vi "shoot boiler.vi"(7 "go":bool, 8 "error out":errorcluster, 11 "RobotDriveDevRef":T1={"DevStatus"={"status"=FALSE, "code"=0, "source"=""}, "Motors[]"=[], "Square Inputs"=FALSE, "Max Output"=1.0}) -> (0 "error out 2":errorcluster, 3 "RobotDriveDevRef 2":T1={"DevStatus"={"status"=FALSE, "code"=0, "source"=""}, "Motors[]"=[], "Square Inputs"=FALSE, "Max Output"=1.0})   [LabVIEW 2016]
uses:
  <vilib>/Rock Robotics/WPI/RobotDrive/WPI_RobotDriveDevRef.ctl
  <vilib>/Rock Robotics/WPI/MotorControl/WPI_MotorControlDeviceRef.ctl
  <vilib>/Rock Robotics/WPI/MotorControl/WPI_MotorControlType.ctl
  <vilib>/Rock Robotics/SystemInterfaces/DIO/FPGA_DIOPWMChannel.ctl
  <vilib>/Rock Robotics/WPI/PWM/WPI_PWMDeadband.ctl
  <vilib>/Rock Robotics/WPI/ThirdParty/CanMotor/TalonSRX/WPI_CANTalonSRX_APIControlMode.ctl
  <vilib>/Rock Robotics/WPI/Relay/WPI_RelayValue.ctl
  Robot Global Data.vi
  <vilib>/Rock Robotics/WPI/RobotDrive/WPI_RobotDriveArcadeDrive_Standard(NoSaturation).vi
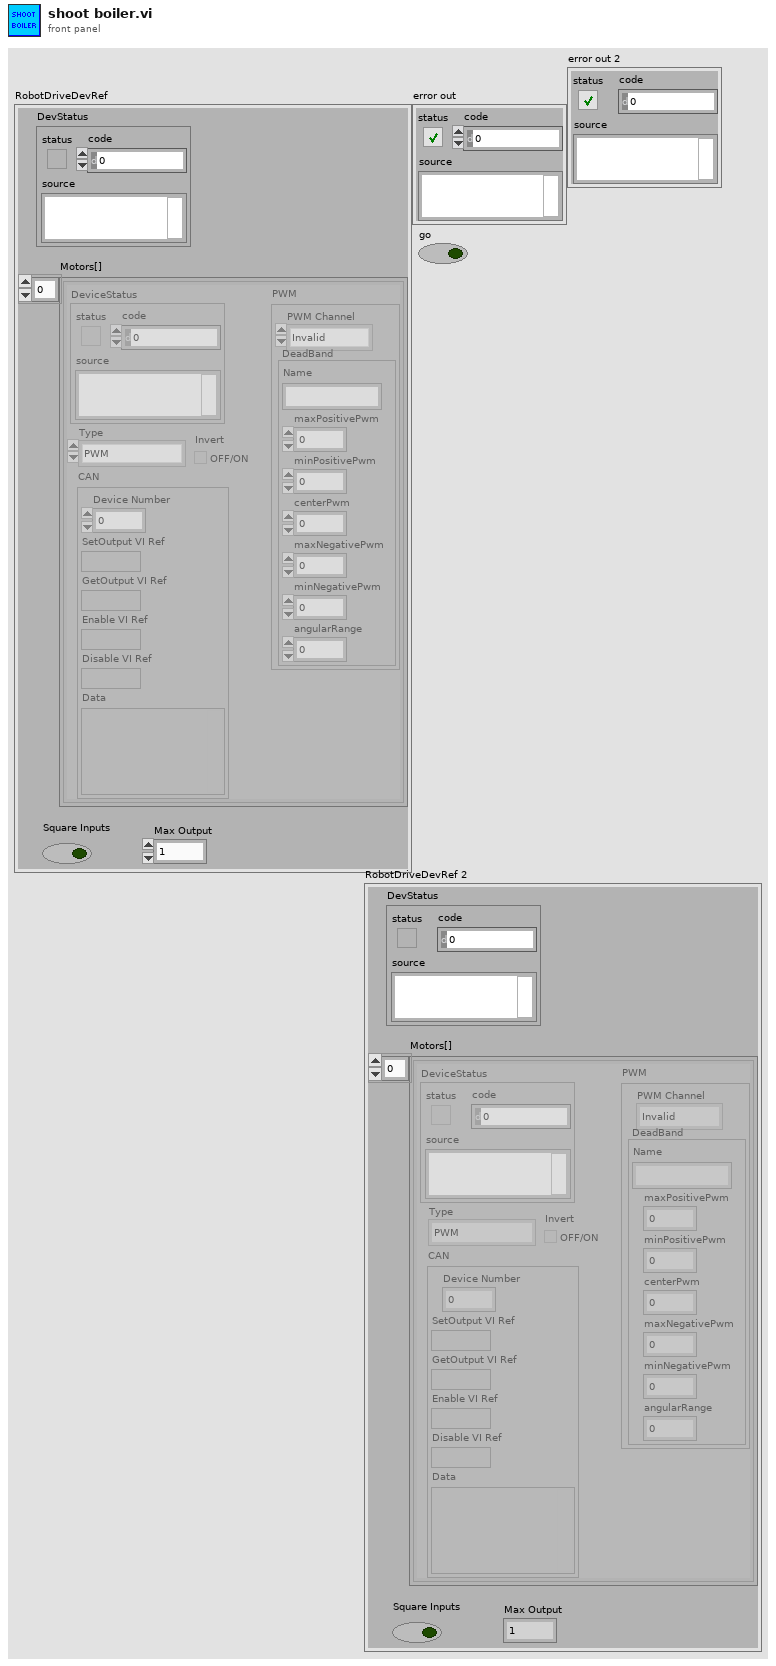
[diagram p1: front panel]
types:
  T1 = typedef "WPI_RobotDriveDevRef.ctl" = cluster{"DevStatus":errorcluster, "Motors[]":T2[], "Square Inputs":bool, "Max Output":dbl}
  T2 = typedef "WPI_MotorControlDeviceRef.ctl" = cluster{"DeviceStatus":errorcluster, "Type":T3, "PWM":cluster{"PWM Channel":T4, "DeadBand":T5}, "CAN":cluster{"Device Number":u8, "SetOutput VI Ref":variant, "GetOutput VI Ref":variant, "Enable VI Ref":variant, "Disable VI Ref":variant, "Data":variant}, "Invert":bool}
  T3 = typedef "WPI_MotorControlType.ctl" = enum16{"PWM", "CAN"}
  T4 = typedef "FPGA_DIOPWMChannel.ctl" = enum8{"PWM 0", "PWM 1", "PWM 2", "PWM 3", "PWM 4", "PWM 5", "PWM 6", "PWM 7", "PWM 8", "PWM 9", "PWM MXP 0", "PWM MXP 1", "PWM MXP 2", "PWM MXP 3", "PWM MXP 4", "PWM MXP 5", "PWM MXP 6", "PWM MXP 7", "PWM MXP 8", "PWM MXP 9", "Invalid"}
  T5 = typedef "WPI_PWMDeadband.ctl" = cluster{"Name":string, "maxPositivePwm":i32, "minPositivePwm":i32, "centerPwm":i32, "maxNegativePwm":i32, "minNegativePwm":i32, "angularRange":u16}
  T6 = typedef "WPI_CANTalonSRX_APIControlMode.ctl" = enum8{"Percent VBus", "Speed", "Position", "Slave", "Unchanged / Invalid", "Voltage Compensation", "Current", "Motion Profile", "Motion Magic"}
  T7 = typedef "WPI_RelayValue.ctl" = enum16{"Off", "On", "Forward", "Reverse"}
  T8 = typedef "WPI_RelayDevRef.ctl" = cluster{"DevStatus":errorcluster, "Relay Channel":T9, "Relay Direction":T10}
  T9 = typedef "FPGA_DIORelayChannel.ctl" = enum8{"Relay 0", "Relay 1", "Relay 2", "Relay 3", "Invalid"}
  T10 = typedef "WPI_RelayDirection.ctl" = enum16{"Both directions", "Forward only", "Reverse only"}
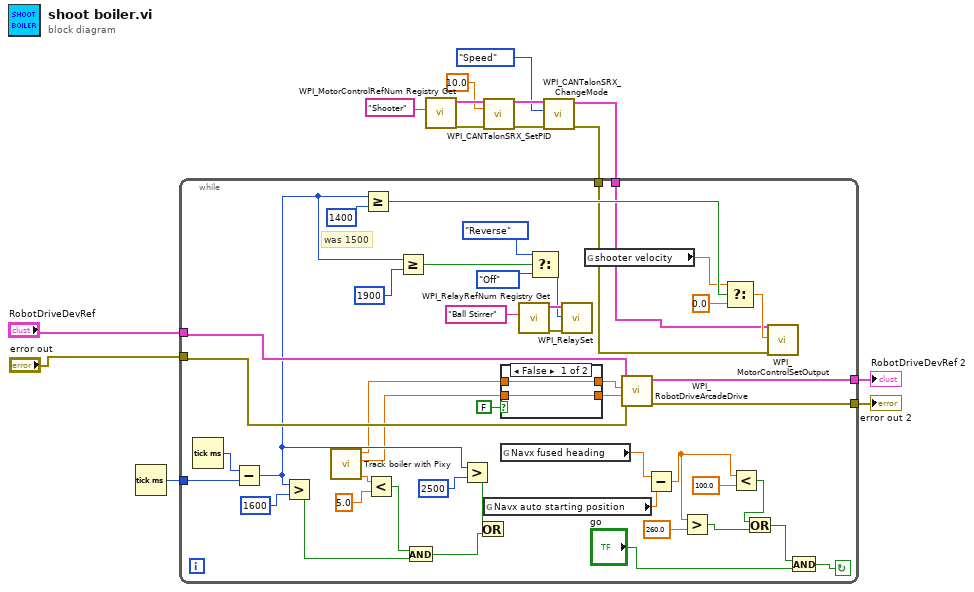
[diagram p0: block diagram]
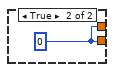
[diagram p2: hidden frame]
diagram:
  n1 = Tick Count (ms)() -> (millisecond timer value=w14:u32)
  n2 = call <vilib>:"WPI_MotorControlRefNum Registry Get.vi"("refnum name"="Shooter") -> ("error out"=w7:errorcluster, "MotorControlDevRef"=w8:T2)  [unwired: 9 in]
  n3 = call <vilib>:"WPI_CANTalonSRX_SetPID.vi"("CAN Talon SRX Ref"=w8, "P"=10.0, "error in (no error)"=w7) -> ("CAN Talon SRX Ref"=w5:T2, "error out"=w4:errorcluster)  [unwired: 11 in]
  n4 = call <vilib>:"WPI_CANTalonSRX_ChangeMode.vi"("error in (no error)"=w4, "Control Mode"=WPI_CANTalonSRX_APIControlMode."Speed", "CAN Talon SRX Ref"=w5) -> ("error out"=w1:errorcluster, "CAN Talon SRX Ref"=w2:T2)  [unwired: 7 in]
  n5 = while {
    tunnel: "RobotDriveDevRef" -> [w54]
    tunnel: "error out" -> [w53]
    tunnel: w14 -> [w57]
    tunnel: [w30] -> w10
    tunnel: [w29] -> w11
    tunnel: w2 -> [w28]
    tunnel: w1 -> [w27]
    stop <- w23 continue-if-true
    # "was 1500"
    n6 = Tick Count (ms)() -> (millisecond timer value=w56:u32)
    n7 = Subtract(x=w56, y=w57) -> (x-y=w49:u32)
    n8 = Greater?(x=w49, y=u32 1600) -> (0:w52:bool)
    n9 = call "Track boiler with Pixy.vi"() -> ("%error"=w59:dbl, "y output"=w43:dbl, "x output"=w45:dbl)  [unwired: 7 in, 1 out]
    n10 = Greater Or Equal?(x=w49, y=u32 1400) -> (x >= y?=w39:bool)
    n11 = Less?(x=w59, y=5.0) -> (x < y?=w51:bool)
    n12 = Greater Or Equal?(x=w49, y=u32 1900) -> (x >= y?=w31:bool)
    n13 = And(x=w51, y=w52) -> (x .and. y?=w47:bool)
    n14 = Greater?(x=w49, y=u32 2500) -> (0:w48:bool)
    n15 = Or(x=w48, y=w47) -> ()  [unwired: 1 out]
    n16 = global read "Robot Global Data.vi" "Navx auto starting position"() -> (w17:dbl)
    n17 = case shown="False" FALSE {
      tunnel: [w61 w62] -> w46
      tunnel: w45 -> [w61 _]
      tunnel: [w60 w62] -> w44
      tunnel: w43 -> [w60 _]
      frame False {
      }
      frame True {
        w62 = 0
      }
    }
    n18 = global read "Robot Global Data.vi" "Navx fused heading"() -> (w16:dbl)
    n19 = call <vilib>:"WPI_RelayRefNum Registry Get.vi"("refnum name"="Ball Stirrer") -> ("error out"=w38:errorcluster, "RelayDevRef"=w37:T8)  [unwired: 9 in]
    n20 = Select(t=WPI_RelayValue."Reverse" ("RelayValue"), s=w31, f=WPI_RelayValue."Off") -> (s? t:f=w33:T7)
    n21 = call <vilib>:"WPI_RelaySet.vi"("error in (no error)"=w38, "RelayValue"=w33, "RelayDevRef"=w37) -> ()  [unwired: 7 in, 2 out]
    n22 = global read "Robot Global Data.vi" "shooter velocity"() -> (w26:dbl)
    n23 = call-poly <vilib>:"WPI_RobotDriveArcadeDrive.vi"("error in (no error)"=w53, "Y axis value"=w44, "X axis value"=w46, "RobotDriveDevRef"=w54) -> ("error out"=w29:errorcluster, "RobotDriveDevRef"=w30:T1)  [unwired: 5 in, 1 out]
    n24 = Subtract(x=w16, y=w17) -> (x-y=w15:dbl)
    n25 = Greater?(x=w15, y=260.0) -> (0:w19:bool)
    n26 = Select(t=w26, s=w39, f=0.0) -> (s? t:f=w40:dbl)
    n27 = Less?(x=w15, y=100.0) -> (x < y?=w21:bool)
    n28 = Or(x=w21, y=w19) -> (x .or. y?=w22:bool)
    n29 = call <vilib>:"WPI_MotorControlSetOutput.vi"("error in (no error)"=w27, "Output"=w40, "MotorControlDevRef"=w28) -> ()  [unwired: 6 in, 3 out]
    n30 = And(x=w22, y="go") -> (x .and. y?=w23:bool)
  }
  "error out 2" <- w11
  "RobotDriveDevRef 2" <- w10
